vi "FRcmd Global.vi"() -> ()   [LabVIEW 2014]
panel:
  out "FRcmd Global":dbl
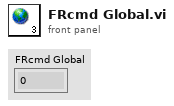
[diagram p1: front panel]
diagram:
